vi "Compute DistanceToTarget2.vi"(8 "Rect":T1, 9 "Camera Type":T3, 10 "Ring":u16(ring) items=["Cube", "Tape", "Switch LED", "Scale LED"], 11 "Image Src":T2) -> (1 "Angles":cluster{"Azimuth":dbl, "Elevation":dbl}, 2 "Distance (ft)":dbl, 3 "Image Dst Out":T2)   [LabVIEW 2017]
doc: "Using the camera lens information and the real world size of the target, use trig and ratios to determine the distance to the target. Also returns the location relative to the image center in a (-1 , 1) coordinate system that may be useful for steering the robot."
uses:
  Camera Types.ctl
  <vilib>/vision/Image Controls.llb/IMAQ Image.ctl
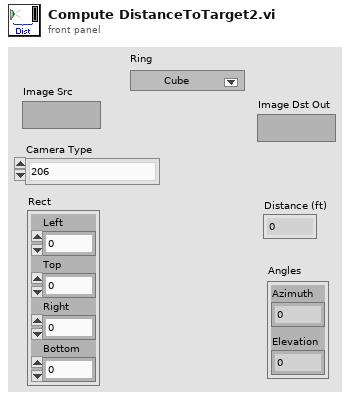
[diagram p1: front panel]
types:
  T1 = cluster{"Left":dbl, "Top":dbl, "Right":dbl, "Bottom":dbl}
  T2 = typedef "IMAQ Image.ctl" = refnum<image>
  T3 = typedef "Camera Types.ctl" = enum16{"206", "1011", "1013", "MS HD3000 square", "MS HD3000 640x480"}
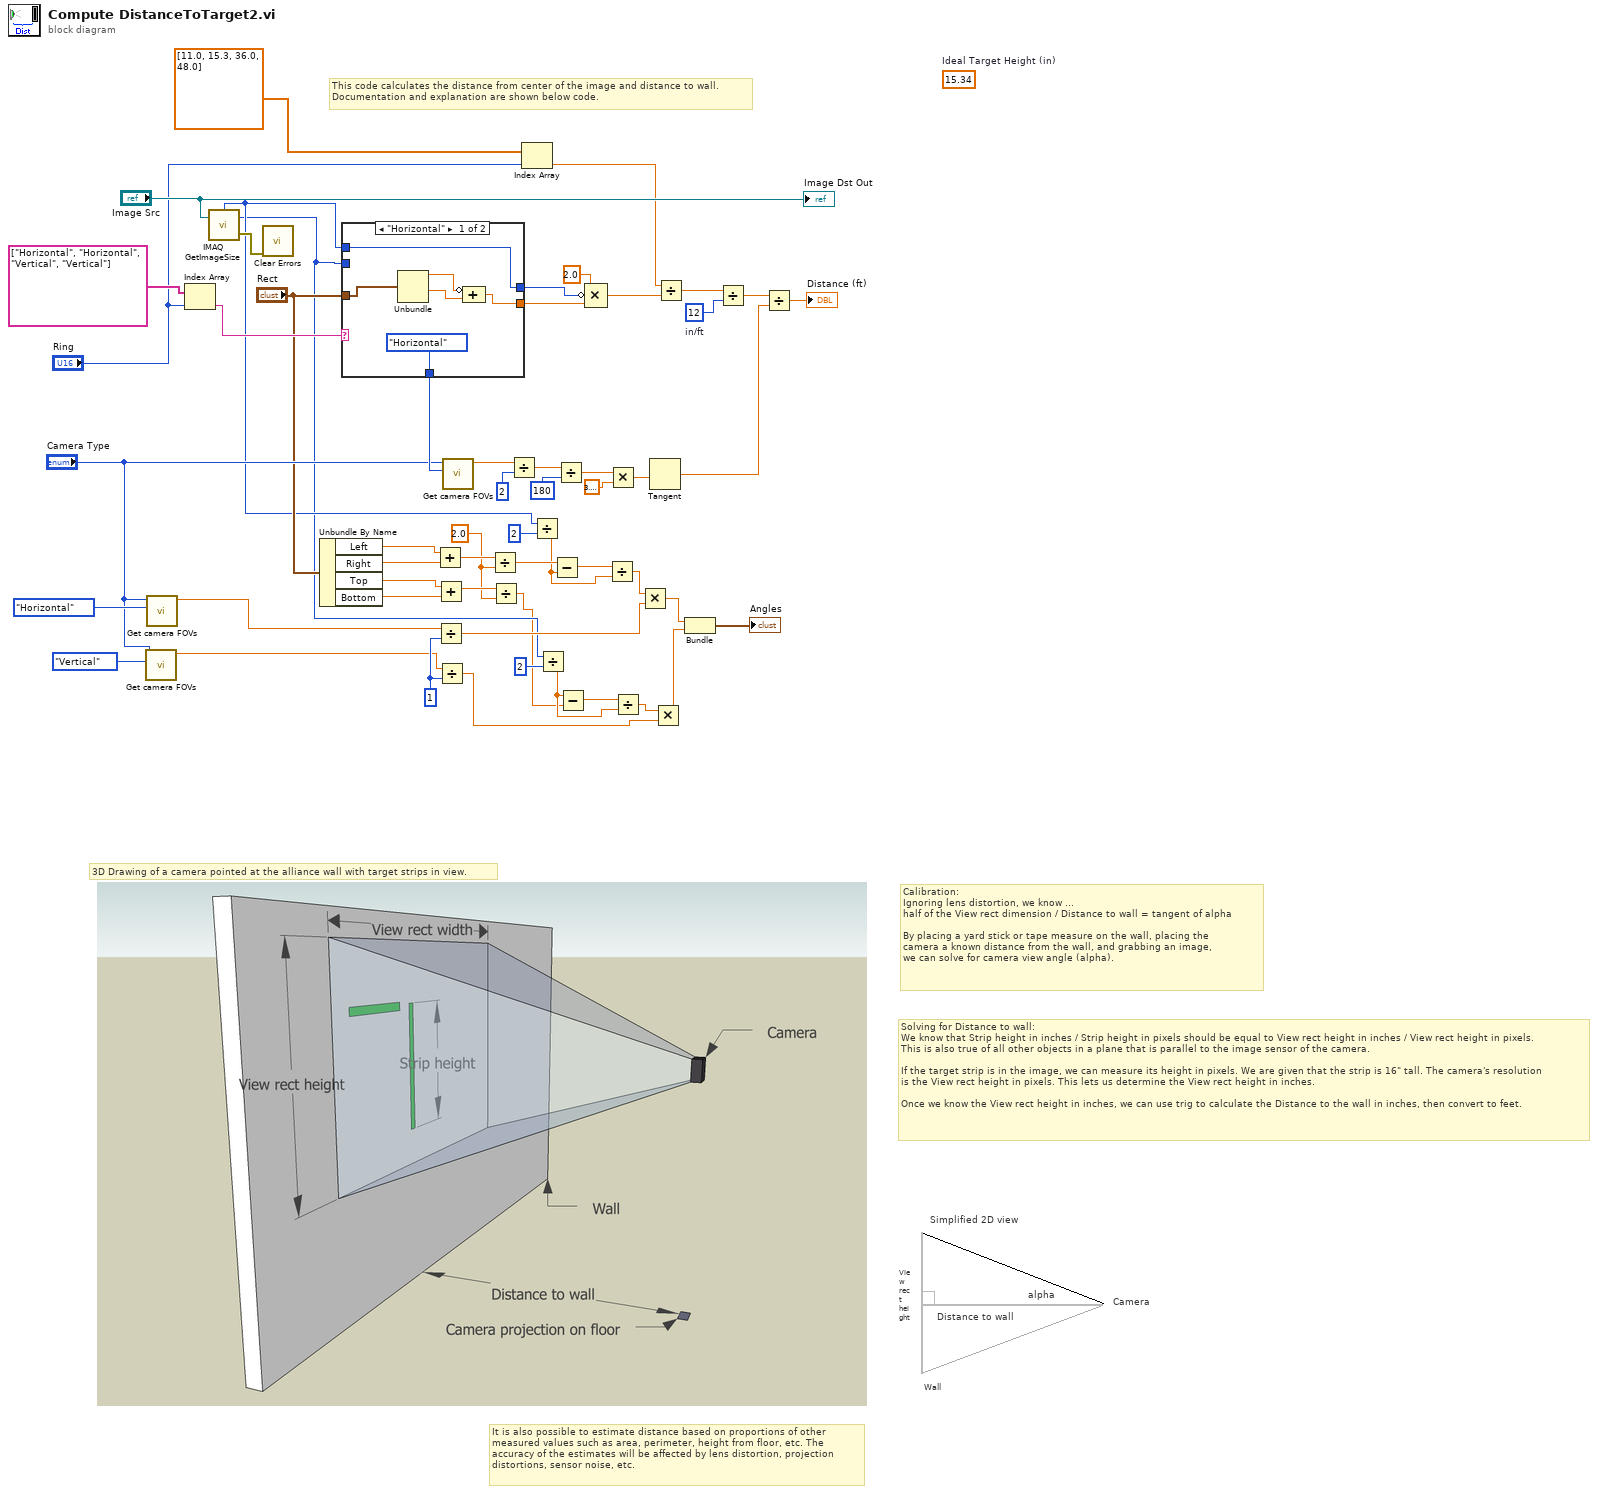
[diagram p0: block diagram]
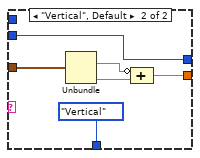
[diagram p2: hidden frame]
diagram:
  w19 = 1
  w20 = 2.0 ("y")
  (unwired) 15.34  # Ideal Target Height (in)
  w49 = 12  # in/ft
  # "It is also possible to estimate distance based on proportions of other\nmeasured values such as area, perimeter, height from floor, etc. The\naccuracy of the estimates will be affected by lens distortion, projection\ndistortions, sensor noise, etc."
  # "Wall"
  # "Camera"
  # "Simplified 2D view"
  # "Solving for Distance to wall:\nWe know that Strip height in inches / Strip height in pixels should be equal to View rect height in inches / View rect height in pixels.\nThis is also true of all other objects in a plane that is parallel to the image sensor of the camera.\n\nIf the target strip is in the image, we can measure its height in pixels. We are given that the strip is 16\" tall. The camera's resolution\nis the View rect height in pixels. This lets us determine the View rect height in inches.\n\nOnce we know the View rect height in inches, we can use trig to calculate the Distance to the wall in inches, then convert to feet."
  # "3D Drawing of a camera pointed at the alliance wall with target strips in view."
  # "Distance to wall"
  # "View rect height"
  # "alpha"
  # "Calibration:\nIgnoring lens distortion, we know ...\nhalf of the View rect dimension / Distance to wall = tangent of alpha\n\nBy placing a yard stick or tape measure on the wall, placing the\ncamera a known distance from the wall, and grabbing an image,\nwe can solve for camera view angle (alpha)."
  # "This code calculates the distance from center of the image and distance to wall.\nDocumentation and explanation are shown below code."
  n1 = call "Get camera FOVs.vi"("Type"=enum16{"Horizontal", "Vertical", "Diagonal"}."Vertical", "Camera Type"="Camera Type") -> ("FOV"=w17:dbl)  [unwired: 8 in, 1 out]
  n2 = call "Get camera FOVs.vi"("Type"=enum16{"Horizontal", "Vertical", "Diagonal"}."Horizontal", "Camera Type"="Camera Type") -> ("FOV"=w18:dbl)  [unwired: 8 in, 1 out]
  n3 = Index Array(array=string[] ["Horizontal", "Horizontal", "Vertical", "Vertical"], index="Ring") -> (element=w35:string)
  n4 = call "IMAQ GetImageSize"("Image"="Image Src") -> ("Y Resolution"=w3:i32, "X Resolution"=w15:i32, "error out"=w43:errorcluster)  [unwired: 3 in]
  n5 = call <vilib>:"Clear Errors.vi"("error in (no error)"=w43) -> ()  [unwired: 5 in, 2 out]
  n6 = Unbundle By Name("Rect") -> ("Left"=w26:dbl, "Right"=w25:dbl, "Top"=w24:dbl, "Bottom"=w23:dbl)
  n7 = case shown="\"Horizontal\"" w35 {
    tunnel: [enum16{"Horizontal", "Vertical", "Diagonal"}."Horizontal" ("Angle") enum16{"Horizontal", "Vertical", "Diagonal"}."Vertical" ("Angle")] -> w42
    tunnel: "Rect" -> [w59 w66]
    tunnel: [w56 w63] -> w40
    tunnel: w3 -> [_ w62]
    tunnel: w15 -> [w61 _]
    tunnel: [w61 w62] -> w37
    frame "Horizontal" {
      n8 = Unbundle(w59) -> ("Left"=w58:dbl, "Right"=w57:dbl)  [unwired: 2 out]
      n9 = Compound Arithmetic op=ADD(invert w58, w57) -> (w56:dbl)
    }
    frame "Vertical", Default {
      n10 = Unbundle(w66) -> ("Top"=w64:dbl, "Bottom"=w65:dbl)  [unwired: 2 out]
      n11 = Compound Arithmetic op=ADD(invert w64, w65) -> (w63:dbl)
    }
  }
  n12 = Add(x=w26, y=w25) -> (x+y=w22:dbl)
  n13 = Add(x=w24, y=w23) -> (x+y=w21:dbl)
  n14 = Divide(x=w18, y=w19) -> (x/y=w10:dbl)
  n15 = Divide(x=w17, y=w19) -> (x/y=w5:dbl)
  n16 = call "Get camera FOVs.vi"("Type"=w42, "Camera Type"="Camera Type") -> ("FOV"=w46:dbl)  [unwired: 8 in, 1 out]
  n17 = Divide(x=w22, y=w20) -> (x/y=w16:dbl)
  n18 = Divide(x=w21, y=w20) -> (x/y=w1:dbl)
  n19 = Divide(x=w46, y=2) -> (x/y=w52:dbl)
  n20 = Index Array(array=dbl[] [11.0, 15.3, 36.0, 48.0], index="Ring") -> (element=w32:dbl)
  n21 = Divide(x=w15, y=2) -> (x/y=w12:dbl)
  n22 = Divide(x=w3, y=2) -> (x/y=w2:dbl)
  n23 = Subtract(x=w16, y=w12) -> (x-y=w13:dbl)
  n24 = Divide(x=w52, y=180) -> (x/y=w51:dbl)
  n25 = Subtract(x=w2, y=w1) -> (x-y=w8:dbl)
  n26 = Compound Arithmetic op=MULTIPLY(2.0, invert w37, w40) -> (w44:dbl)
  n27 = Divide(x=w13, y=w12) -> (x/y=w11:dbl)
  n28 = Multiply(x=w51, y=3.141592653589793) -> (x*y=w53:dbl)
  n29 = Divide(x=w8, y=w2) -> (x/y=w6:dbl)
  n30 = Multiply(x=w11, y=w10) -> (x*y=w9:dbl)
  n31 = Tangent(1:w53) -> (0:w48:dbl)
  n32 = Multiply(x=w6, y=w5) -> (x*y=w4:dbl)
  n33 = Divide(x=w32, y=w44) -> (x/y=w38:dbl)
  n34 = Bundle(w9, w4) -> (→"Angles":cluster{dbl, dbl})  [unwired: 1 in]
  n35 = Divide(x=w38, y=w49) -> (x/y=w47:dbl)
  n36 = Divide(x=w47, y=w48) -> (x/y=→"Distance (ft)":dbl)
  "Image Dst Out" <- "Image Src"
